vi "CRYHarmonics array order.vi"(10 "Type":u16, 11 "Harmonics array in":dbl[](array[numeric]) format="%.2f") -> (2 "Make Fundamental curve?":bool, 3 "Harmonics array out":dbl[](array[numeric]) format="%.2f")   [LabVIEW 2013]
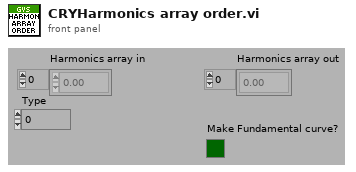
[diagram p1: front panel]
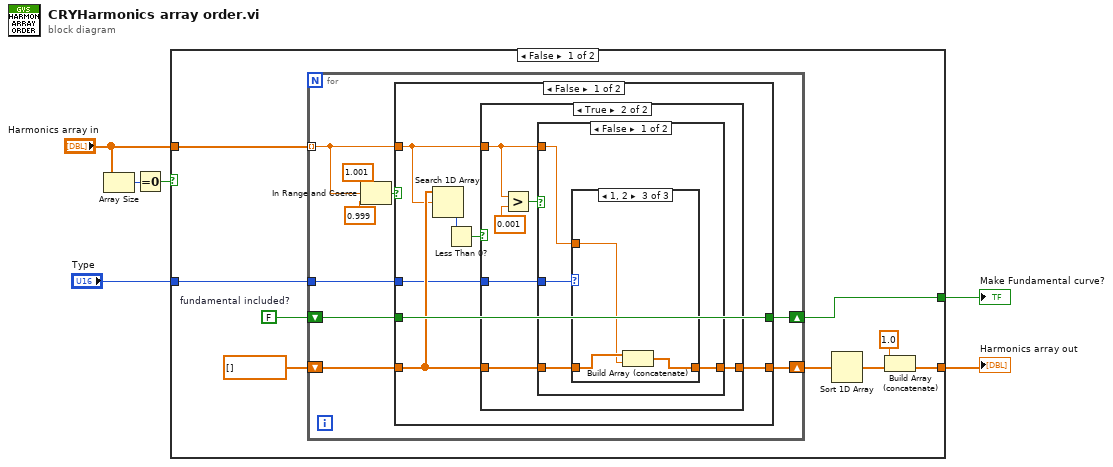
[diagram p0: block diagram]
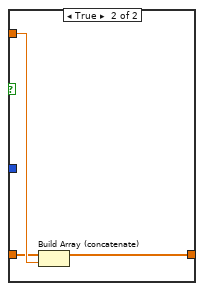
[diagram p5: hidden frame]
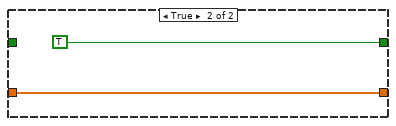
[diagram p6: hidden frame]
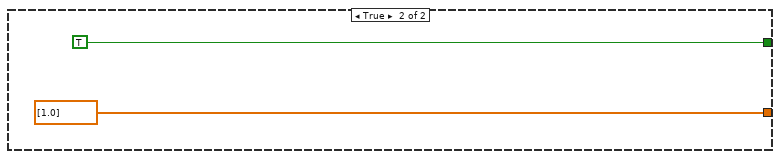
[diagram p7: hidden frame]
diagram:
  n1 = Array Size(array="Harmonics array in") -> (size(s)=w4:i32)
  n2 = Equal To 0?(x=w4) -> (x = 0?=w2:bool)
  n3 = case shown="False" w2 {
    tunnel: "Harmonics array in" -> [w15 _]
    tunnel: [w10 dbl[] [1.0]] -> w6
    tunnel: [w8 TRUE ("fundamental included?")] -> w5
    tunnel: "Type" -> [w7 _]
    frame False {
      w14 = FALSE  # fundamental included?
      n4 = for {
        tunnel: w15 -> [w17] mode=indexing
        shift-right: [w18] -> w8
        shift-left: w14 -> [w19]
        shift-right: [w20] -> w12
        shift-left: dbl[] [] ("Harmonics array in") -> [w21]
        tunnel: w7 -> [w16]
        n5 = In Range and Coerce(upper limit=1.001, x=w17, lower limit=0.999) -> (In Range?=w22:bool)  [unwired: 1 out]
        n6 = case shown="False" w22 {
          tunnel: w21 -> [w28 w51]
          tunnel: [w27 w51] -> w20
          tunnel: [w31 TRUE ("fundamental included?")] -> w18
          tunnel: w19 -> [w31 _]
          tunnel: w17 -> [w26 _]
          tunnel: w16 -> [w25 _]
          frame False {
            n7 = Search 1D Array(1D array=w28, element=w26) -> (index of element=w30:i32)  [unwired: 1 out]
            n8 = Less Than 0?(x=w30) -> (x < 0?=w29:bool)
            n9 = case shown="True" w29 {
              tunnel: w28 -> [w32 w35]
              tunnel: [w32 w34] -> w27
              tunnel: w26 -> [_ w36]
              tunnel: w25 -> [_ w33]
              frame False {
              }
              frame True {
                n10 = Greater?(x=w36, y=0.001) -> (0:w37:bool)
                n11 = case shown="False" w37 {
                  tunnel: w36 -> [w39 w49]
                  tunnel: w35 -> [w42 w48]
                  tunnel: [w41 w47] -> w34
                  tunnel: w33 -> [w40 _]
                  frame False {
                    n12 = case shown="1, 2" w40 {
                      tunnel: w42 -> [_ w43 w46]
                      tunnel: [_ w43 w44] -> w41
                      tunnel: w39 -> [_ _ w45]
                      frame Default {
                      }
                      frame 0 {
                      }
                      frame 1, 2 {
                        n13 = Build Array (concatenate)(w46, w45) -> (w44:dbl[])
                      }
                    }
                  }
                  frame True {
                    n14 = Build Array (concatenate)(w48, w49) -> (w47:dbl[])
                  }
                }
              }
            }
          }
          frame True {
          }
        }
      }
      n15 = Sort 1D Array(array=w12) -> (sorted array=w11:dbl[])
      n16 = Build Array (concatenate)(1.0, w11) -> (w10:dbl[])
    }
    frame True {
    }
  }
  "Harmonics array out" <- w6
  "Make Fundamental curve?" <- w5
